vi "Init.vi"(7 "SequenceCountService":refnum<class "SequenceCountService.lvclass">, 8 "error in (no error)":errorcluster, 10 "Node":refnum<class "Node Config.lvclass">) -> (0 "error out":errorcluster, 3 "DiscoveryService out":refnum<class "NodeDiscovery.lvclass">)   [LabVIEW 2020, in "Vecto.lvlib" / "NodeDiscovery.lvclass"]
uses:
  NodeDiscovery.lvclass
  Node Config/Node Config.lvclass
  SequenceCountService/SequenceCountService.lvclass
  proto/Discovery/Data.ctl
  proto/Service/Data.ctl
  proto/ServiceType/Enumeration.ctl
  NodeDiscovery.lvclass/NodeDiscovery.ctl
  proto/ServiceType/ServiceType.lvlib
  proto/Service/Service.lvlib
  proto/Discovery/Discovery.lvlib
panel:
  in  "Advertise":bool
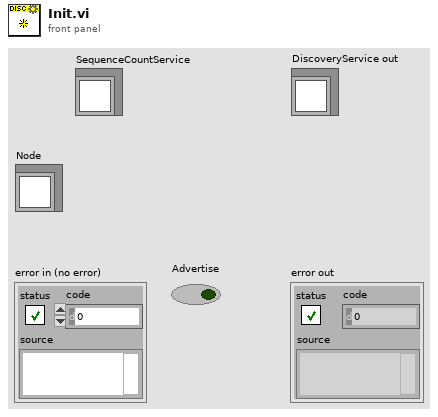
[diagram p1: front panel]
types:
  T1 = typedef "Discovery.lvlib/Data.ctl" = cluster{"node_id":u32, "name":string, "ip":u32, "status":string, "services":T2[], "system":string, "cluster":string}
  T2 = typedef "Service.lvlib/Data.ctl" = cluster{"type":T3, "port":i32}
  T3 = typedef "ServiceType.lvlib/Enumeration.ctl" = enum16{"SERVICETYPE_UNKNOWN", "SERVICETYPE_TCPSERVER", "SERVICETYPE_HTTPSERVER"}
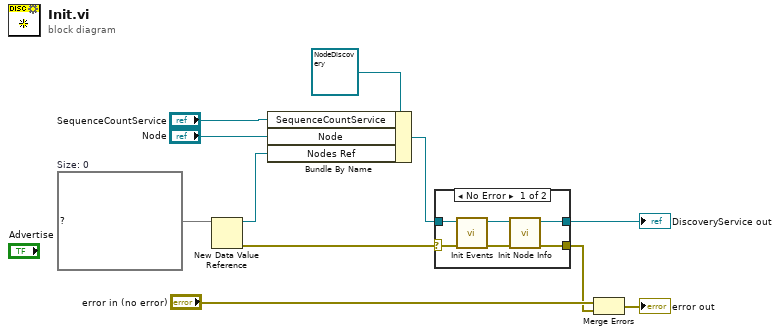
[diagram p0: block diagram]
diagram:
  w9 = map{u32, T1} {}  # Size: 0
  n1 = New Data Value Reference(data value=w9) -> (data value reference=w8:refnum<data-value>, error out=w5:errorcluster)  [unwired: 1 in]
  n2 = Bundle By Name(cluster=refnum<class "NodeDiscovery.lvclass"> refnum ("DiscoveryService in"), "SequenceCountService"="SequenceCountService", "Node"="Node", "Nodes Ref"=w8) -> (w7:refnum<class "NodeDiscovery.lvclass">)
  n3 = case shown="No Error" w5 {
    selector: w5 -> [w16 w18]
    tunnel: w7 -> [w17 w19]
    tunnel: [w12 w19] -> w6
    tunnel: [w14 w18] -> w2
    frame No Error {
      n4 = call "Init Events.vi"("error in (no error)"=w16, "DiscoveryService in"=w17) -> ("error out"=w15:errorcluster, "DiscoveryService out"=w13:refnum<class "NodeDiscovery.lvclass">)  [unwired: 8 in]
      n5 = call "Init Node Info.vi"("error in (no error)"=w15, "DiscoveryService in"=w13) -> ("error out"=w14:errorcluster, "DiscoveryService out"=w12:refnum<class "NodeDiscovery.lvclass">)  [unwired: 8 in]
    }
    frame Error {
    }
  }
  "DiscoveryService out" <- w6
  n6 = Merge Errors("error in (no error)", w2) -> (→"error out":errorcluster)
